vi "Node_ID_AlarmErrors.vi"(11 "error in":errorcluster) -> (4 "transposed array":string[][](array[string]), 6 "Node ID":string[](array[string]), 10 "Name":string[](array[string]), 12 "node RU":T1[](array[typedef]), 13 "node RU 2":T1[](array[typedef]), 14 "node RU 3":string[](array[string]), 15 "error out":errorcluster)   [LabVIEW 2019]
uses:
  <vilib>/OPCUA/controls/NodeId.ctl
panel:
  out "output array":T1[](array[typedef])
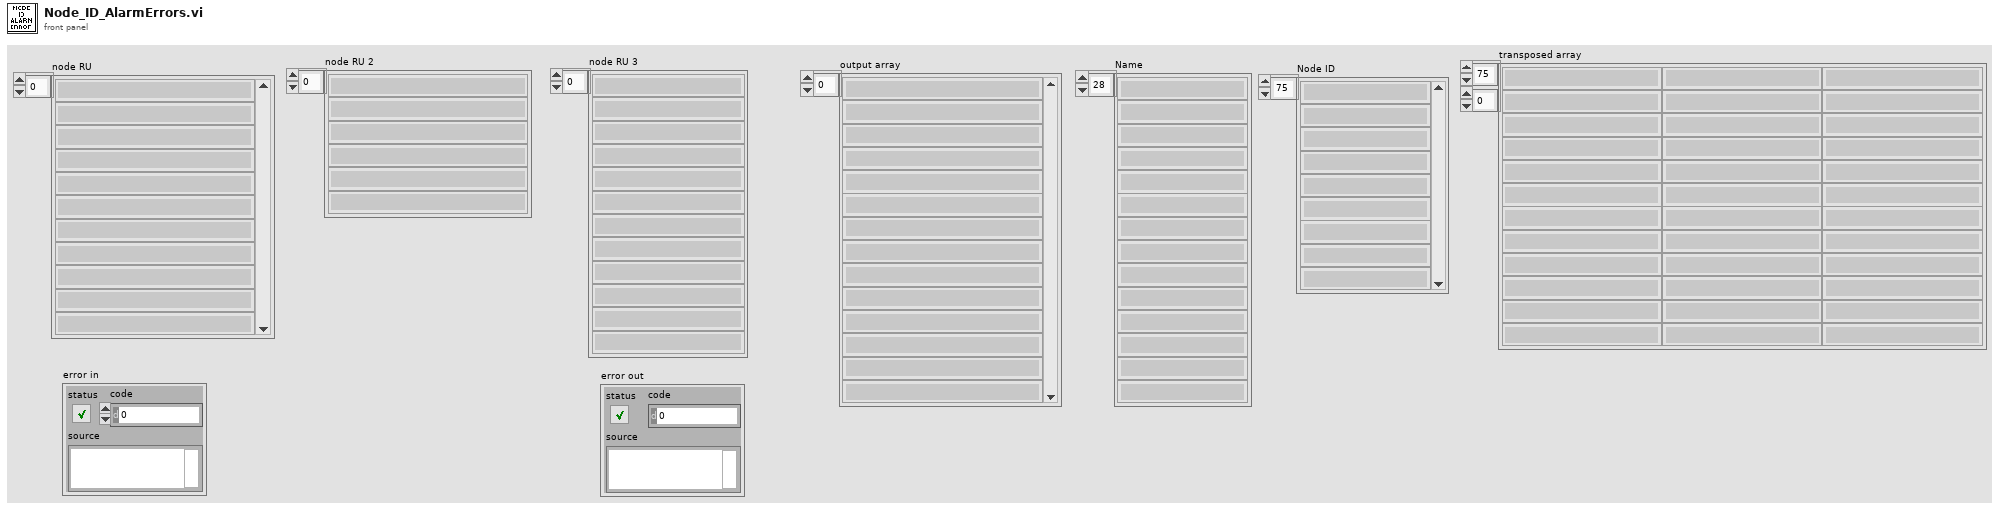
[diagram p1: front panel]
types:
  T1 = typedef "NodeId.ctl" = string
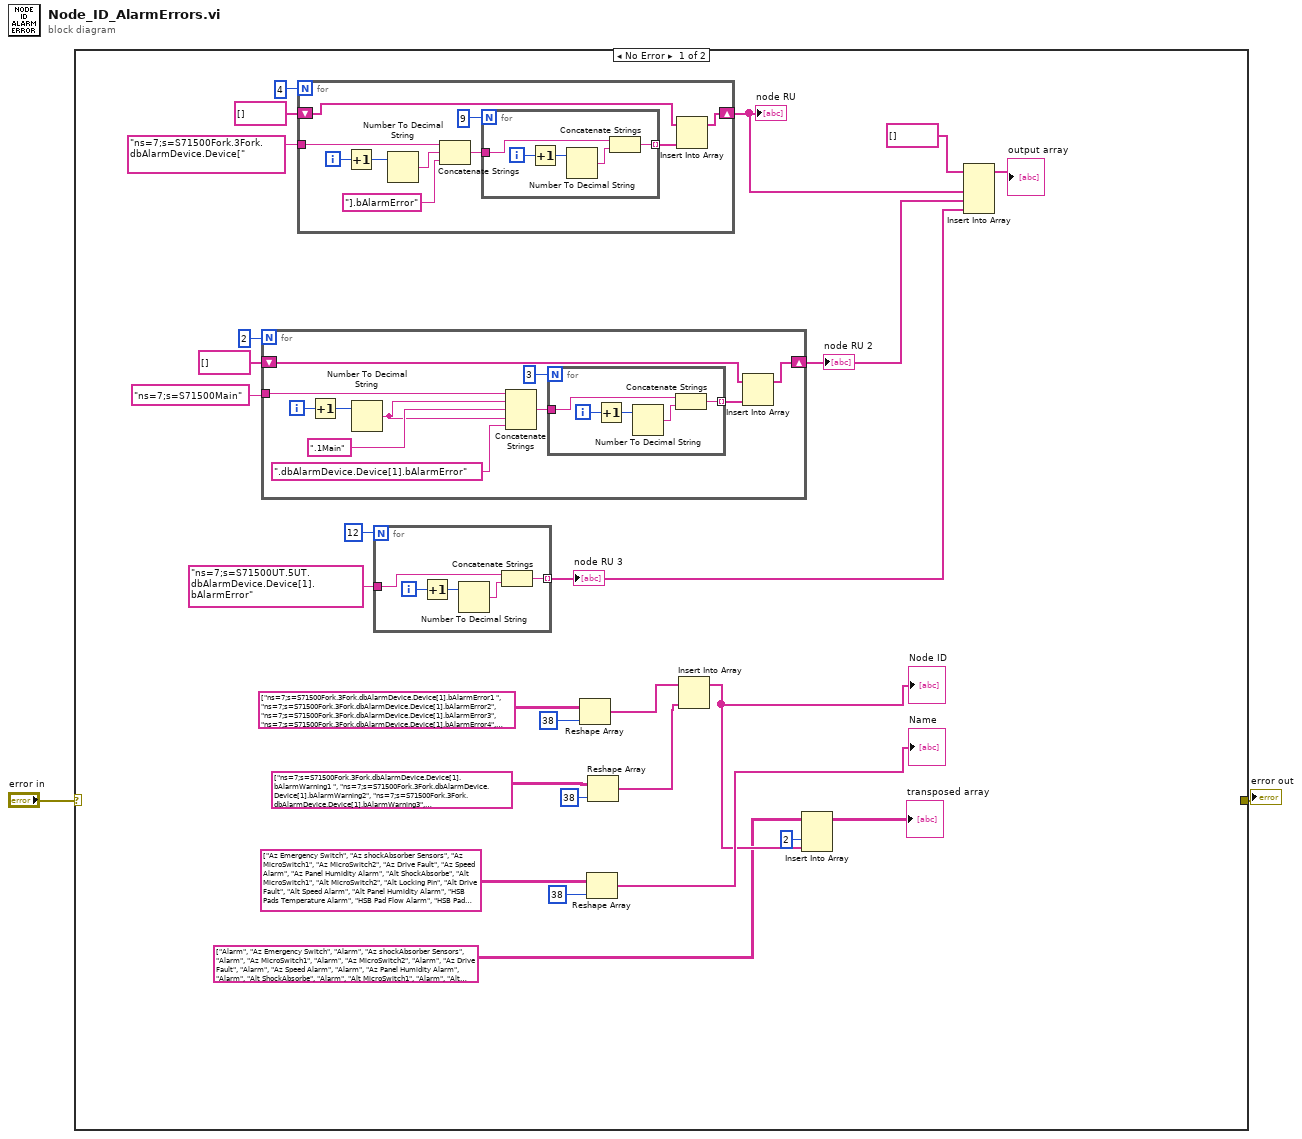
[diagram p0: block diagram]
diagram:
  n1 = case shown="No Error" "error in" {
    selector: "error in" -> [_ w65]
    tunnel: [_ w65] -> w1
    frame No Error {
      n2 = for {
        N: 2 -> [_]
        tunnel: T1 "ns=7;s=S71500Main" ("node RU") -> [w43]
        shift-right: [w40] -> w18
        shift-left: T1[] [] ("node RU") -> [w38]
        i -> [w42]
        n3 = Increment(x=w42) -> (x+1=w44:i32)
        n4 = Number To Decimal String(number=w44) -> (decimal integer string=w36:string)  [unwired: 1 in]
        n5 = Concatenate Strings(w43, w36, ".1Main" ("string"), w36, ".dbAlarmDevice.Device[1].bAlarmError" ("string")) -> (w41:string)
        n6 = for {
          N: 3 -> [_]
          tunnel: w41 -> [w49]
          tunnel: [w45] -> w39 mode=indexing
          i -> [w48]
          n7 = Increment(x=w48) -> (x+1=w47:i32)
          n8 = Number To Decimal String(number=w47) -> (decimal integer string=w46:string)  [unwired: 1 in]
          n9 = Concatenate Strings(w49, w46) -> (w45:string)
        }
        n10 = Insert Into Array(array=w38, new element=w39) -> (w40:T1[])  [unwired: 1 in]
      }
      "node RU 2" <- w18
      n11 = for {
        N: 4 -> [_]
        tunnel: T1 "ns=7;s=S71500Fork.3Fork.dbAlarmDevice.Device[" ("node RU") -> [w57]
        shift-right: [w52] -> w19
        shift-left: T1[] [] ("node RU") -> [w50]
        i -> [w56]
        n12 = Increment(x=w56) -> (x+1=w59:i32)
        n13 = Number To Decimal String(number=w59) -> (decimal integer string=w58:string)  [unwired: 1 in]
        n14 = Concatenate Strings(w57, w58, "].bAlarmError" ("string")) -> (w53:string)
        n15 = for {
          N: 9 -> [_]
          tunnel: w53 -> [w64]
          tunnel: [w60] -> w51 mode=indexing
          i -> [w63]
          n16 = Increment(x=w63) -> (x+1=w62:i32)
          n17 = Number To Decimal String(number=w62) -> (decimal integer string=w61:string)  [unwired: 1 in]
          n18 = Concatenate Strings(w64, w61) -> (w60:string)
        }
        n19 = Insert Into Array(array=w50, new element=w51) -> (w52:T1[])  [unwired: 1 in]
      }
      "node RU" <- w19
      n20 = for {
        N: 12 -> [_]
        tunnel: T1 "ns=7;s=S71500UT.5UT.dbAlarmDevice.Device[1].bAlarmError" ("node RU") -> [w33]
        tunnel: [w29] -> w17 mode=indexing
        i -> [w32]
        n21 = Increment(x=w32) -> (x+1=w31:i32)
        n22 = Number To Decimal String(number=w31) -> (decimal integer string=w30:string)  [unwired: 1 in]
        n23 = Concatenate Strings(w33, w30) -> (w29:string)
      }
      "node RU 3" <- w17
      n24 = Reshape Array(string[][] [["ns=7;s=S71500Fork.3Fork.dbAlarmDevice.Device[1].bAlarmError1 "], ["ns=7;s=S71500Fork.3Fork.dbAlarmDevice.Device[1].bAlarmError2"], ["ns=7;s=S71500Fork.3Fork.dbAlarmDevice.Device[1].bAlarmError3"], ["ns=7;s=S71500Fork.3Fork.dbAlarmDevice.Device[1].bAlarmError4"], ["ns=7;s=S71500Fork.3Fork.dbAlarmDevice.Device[1].bAlarmError6"], ["ns=7;s=S71500Fork.3Fork.dbAlarmDevice.Device[1].bAlarmError7"], ["ns=7;s=S71500Fork.3Fork.dbAlarmDevice.Device[1].bAlarmError8"], ["ns=7;s=S71500Fork.3Fork.dbAlarmDevice.Device[2].bAlarmError2"], ["ns=7;s=S71500Fork.3Fork.dbAlarmDevice.Device[2].bAlarmError3"], ["ns=7;s=S71500Fork.3Fork.dbAlarmDevice.Device[2].bAlarmError4"], ["ns=7;s=S71500Fork.3Fork.dbAlarmDevice.Device[2].bAlarmError5"], ["ns=7;s=S71500Fork.3Fork.dbAlarmDevice.Device[2].bAlarmError6"], ["ns=7;s=S71500Fork.3Fork.dbAlarmDevice.Device[2].bAlarmError7"], ["ns=7;s=S71500Fork.3Fork.dbAlarmDevice.Device[2].bAlarmError8"], ["ns=7;s=S71500Fork.3Fork.dbAlarmDevice.Device[3].bAlarmError2"], ["ns=7;s=S71500Fork.3Fork.dbAlarmDevice.Device[3].bAlarmError3"], ["ns=7;s=S71500Fork.3Fork.dbAlarmDevice.Device[3].bAlarmError4"], ["ns=7;s=S71500Fork.3Fork.dbAlarmDevice.Device[3].bAlarmError5"], ["ns=7;s=S71500Fork.3Fork.dbAlarmDevice.Device[4].bAlarmError8"], ["ns=7;s=S71500Fork.3Fork.dbAlarmDevice.Device[4].bAlarmError9"], ["ns=7;s=S71500Main1.1Main1.dbAlarmDevice.Device[1].bAlarmError1 "], ["ns=7;s=S71500Main1.1Main1.dbAlarmDevice.Device[1].bAlarmError2"], ["ns=7;s=S71500Main1.1Main1.dbAlarmDevice.Device[1].bAlarmError3"], ["ns=7;s=S71500Main2.1Main2.dbAlarmDevice.Device[1].bAlarmError1 "], ["ns=7;s=S71500Main2.1Main2.dbAlarmDevice.Device[1].bAlarmError2"], ["ns=7;s=S71500Main2.1Main2.dbAlarmDevice.Device[1].bAlarmError3"], ["ns=7;s=S71500UT.5UT.dbAlarmDevice.Device[1].bAlarmError1"], ["ns=7;s=S71500UT.5UT.dbAlarmDevice.Device[1].bAlarmError2"], ["ns=7;s=S71500UT.5UT.dbAlarmDevice.Device[1].bAlarmError3"], ["ns=7;s=S71500UT.5UT.dbAlarmDevice.Device[1].bAlarmError4"], ["ns=7;s=S71500UT.5UT.dbAlarmDevice.Device[1].bAlarmError5"], ["ns=7;s=S71500UT.5UT.dbAlarmDevice.Device[1].bAlarmError6"], ["ns=7;s=S71500UT.5UT.dbAlarmDevice.Device[1].bAlarmError7"], ["ns=7;s=S71500UT.5UT.dbAlarmDevice.Device[1].bAlarmError8"], ["ns=7;s=S71500UT.5UT.dbAlarmDevice.Device[1].bAlarmError9"], ["ns=7;s=S71500UT.5UT.dbAlarmDevice.Device[1].bAlarmError10"], ["ns=7;s=S71500UT.5UT.dbAlarmDevice.Device[1].bAlarmError11"], ["ns=7;s=S71500UT.5UT.dbAlarmDevice.Device[1].bAlarmError12"]] ("data"), 38 ("dimension size")) -> (w6:string[])
      n25 = Reshape Array(string[][] [["Az Emergency Switch"], ["Az shockAbsorber Sensors"], ["Az MicroSwitch1"], ["Az MicroSwitch2"], ["Az Drive Fault"], ["Az Speed Alarm"], ["Az Panel Humidity Alarm"], ["Alt ShockAbsorbe"], ["Alt MicroSwitch1"], ["Alt MicroSwitch2"], ["Alt Locking Pin"], ["Alt Drive Fault"], ["Alt Speed Alarm"], ["Alt Panel Humidity Alarm"], ["HSB Pads Temperature Alarm"], ["HSB Pad Flow Alarm"], ["HSB Pad Pressure Alarm"], ["HSB Pads Filters Alarm"], ["Fork Panel Humidity Alarm"], ["Fork Panel Temperator Alarm"], ["Main Emergency Microswitch"], ["UPS Input Alarm"], ["UPS Output Alarm"], ["Main Emergency Microswitch"], ["UPS Input Alarm"], ["UPS Output Alarm"], ["HSB Emergency Alarm"], ["Feed Over Pressure Alarm"], ["Accumulator Pressure Alarm"], ["Main And Reserve Pressure Alarm"], ["HSB Pad Inside Pressure Alarm"], ["HSB Filter Alarm"], ["Oil Level Alarm"], ["Pressure Switch Alarm"], ["Feeds Alarm"], ["UT Panel Humidity Alarm"], ["UT Panel Temperator Alarm"], ["Feed Under Pressure Alarm"]] ("data"), 38 ("dimension size")) -> (→"Name":string[])
      n26 = Reshape Array(string[][] [["ns=7;s=S71500Fork.3Fork.dbAlarmDevice.Device[1].bAlarmWarning1 "], ["ns=7;s=S71500Fork.3Fork.dbAlarmDevice.Device[1].bAlarmWarning2"], ["ns=7;s=S71500Fork.3Fork.dbAlarmDevice.Device[1].bAlarmWarning3"], ["ns=7;s=S71500Fork.3Fork.dbAlarmDevice.Device[1].bAlarmWarning4"], ["ns=7;s=S71500Fork.3Fork.dbAlarmDevice.Device[1].bAlarmWarning6"], ["ns=7;s=S71500Fork.3Fork.dbAlarmDevice.Device[1].bAlarmWarning7"], ["ns=7;s=S71500Fork.3Fork.dbAlarmDevice.Device[1].bAlarmWarning8"], ["ns=7;s=S71500Fork.3Fork.dbAlarmDevice.Device[2].bAlarmWarning2"], ["ns=7;s=S71500Fork.3Fork.dbAlarmDevice.Device[2].bAlarmWarning3"], ["ns=7;s=S71500Fork.3Fork.dbAlarmDevice.Device[2].bAlarmWarning4"], ["ns=7;s=S71500Fork.3Fork.dbAlarmDevice.Device[2].bAlarmWarning5"], ["ns=7;s=S71500Fork.3Fork.dbAlarmDevice.Device[2].bAlarmWarning6"], ["ns=7;s=S71500Fork.3Fork.dbAlarmDevice.Device[2].bAlarmWarning7"], ["ns=7;s=S71500Fork.3Fork.dbAlarmDevice.Device[2].bAlarmWarning8"], ["ns=7;s=S71500Fork.3Fork.dbAlarmDevice.Device[3].bAlarmWarning2"], ["ns=7;s=S71500Fork.3Fork.dbAlarmDevice.Device[3].bAlarmWarning3"], ["ns=7;s=S71500Fork.3Fork.dbAlarmDevice.Device[3].bAlarmWarning4"], ["ns=7;s=S71500Fork.3Fork.dbAlarmDevice.Device[3].bAlarmWarning5"], ["ns=7;s=S71500Fork.3Fork.dbAlarmDevice.Device[4].bAlarmWarning8"], ["ns=7;s=S71500Fork.3Fork.dbAlarmDevice.Device[4].bAlarmWarning9"], ["ns=7;s=S71500Main1.1Main1.dbAlarmDevice.Device[1].bAlarmWarning1 "], ["ns=7;s=S71500Main1.1Main1.dbAlarmDevice.Device[1].bAlarmWarning2"], ["ns=7;s=S71500Main1.1Main1.dbAlarmDevice.Device[1].bAlarmWarning3"], ["ns=7;s=S71500Main2.1Main2.dbAlarmDevice.Device[1].bAlarmWarning1 "], ["ns=7;s=S71500Main2.1Main2.dbAlarmDevice.Device[1].bAlarmWarning2"], ["ns=7;s=S71500Main2.1Main2.dbAlarmDevice.Device[1].bAlarmWarning3"], ["ns=7;s=S71500UT.5UT.dbAlarmDevice.Device[1].bAlarmWarning1"], ["ns=7;s=S71500UT.5UT.dbAlarmDevice.Device[1].bAlarmWarning2"], ["ns=7;s=S71500UT.5UT.dbAlarmDevice.Device[1].bAlarmWarning3"], ["ns=7;s=S71500UT.5UT.dbAlarmDevice.Device[1].bAlarmWarning4"], ["ns=7;s=S71500UT.5UT.dbAlarmDevice.Device[1].bAlarmWarning5"], ["ns=7;s=S71500UT.5UT.dbAlarmDevice.Device[1].bAlarmWarning6"], ["ns=7;s=S71500UT.5UT.dbAlarmDevice.Device[1].bAlarmWarning7"], ["ns=7;s=S71500UT.5UT.dbAlarmDevice.Device[1].bAlarmWarning8"], ["ns=7;s=S71500UT.5UT.dbAlarmDevice.Device[1].bAlarmWarning9"], ["ns=7;s=S71500UT.5UT.dbAlarmDevice.Device[1].bAlarmWarning10"], ["ns=7;s=S71500UT.5UT.dbAlarmDevice.Device[1].bAlarmWarning11"], ["ns=7;s=S71500UT.5UT.dbAlarmDevice.Device[1].bAlarmWarning12"]] ("data"), 38 ("dimension size")) -> (w5:string[])
      n27 = Insert Into Array(array=w6, new element=w5) -> (w4:string[])  [unwired: 1 in]
      "Node ID" <- w4
      n28 = Insert Into Array(array=string[][] [["Alarm", "Az Emergency Switch"], ["Alarm", "Az shockAbsorber Sensors"], ["Alarm", "Az MicroSwitch1"], ["Alarm", "Az MicroSwitch2"], ["Alarm", "Az Drive Fault"], ["Alarm", "Az Speed Alarm"], ["Alarm", "Az Panel Humidity Alarm"], ["Alarm", "Alt ShockAbsorbe"], ["Alarm", "Alt MicroSwitch1"], ["Alarm", "Alt MicroSwitch2"], ["Alarm", "Alt Locking Pin"], ["Alarm", "Alt Drive Fault"], ["Alarm", "Alt Speed Alarm"], ["Alarm", "Alt Panel Humidity Alarm"], ["Alarm", "HSB Pads Temperature Alarm"], ["Alarm", "HSB Pad Flow Alarm"], ["Alarm", "HSB Pad Pressure Alarm"], ["Alarm", "HSB Pads Filters Alarm"], ["Alarm", "Fork Panel Humidity Alarm"], ["Alarm", "Fork Panel Temperator Alarm"], ["Alarm", "Main Emergency Microswitch"], ["Alarm", "UPS Input Alarm"], ["Alarm", "UPS Output Alarm"], ["Alarm", "Main Emergency Microswitch"], ["Alarm", "UPS Input Alarm"], ["Alarm", "UPS Output Alarm"], ["Alarm", "HSB Emergency Alarm"], ["Alarm", "Feed Over Pressure Alarm"], ["Alarm", "Accumulator Pressure Alarm"], ["Alarm", "Main And Reserve Pressure Alarm"], ["Alarm", "HSB Pad Inside Pressure Alarm"], ["Alarm", "HSB Filter Alarm"], ["Alarm", "Oil Level Alarm"], ["Alarm", "Pressure Switch Alarm"], ["Alarm", "Feeds Alarm"], ["Alarm", "UT Panel Humidity Alarm"], ["Alarm", "UT Panel Temperator Alarm"], ["Alarm", "Feed Under Pressure Alarm"], ["Warning", "Az Emergency Switch"], ["Warning", "Az shockAbsorber Sensors"], ["Warning", "Az MicroSwitch1"], ["Warning", "Az MicroSwitch2"], ["Warning", "Az Drive Fault"], ["Warning", "Az Speed Alarm"], ["Warning", "Az Panel Humidity Alarm"], ["Warning", "Alt ShockAbsorbe"], ["Warning", "Alt MicroSwitch1"], ["Warning", "Alt MicroSwitch2"], ["Warning", "Alt Locking Pin"], ["Warning", "Alt Drive Fault"], ["Warning", "Alt Speed Alarm"], ["Warning", "Alt Panel Humidity Alarm"], ["Warning", "HSB Pads Temperature Alarm"], ["Warning", "HSB Pad Flow Alarm"], ["Warning", "HSB Pad Pressure Alarm"], ["Warning", "HSB Pads Filters Alarm"], ["Warning", "Fork Panel Humidity Alarm"], ["Warning", "Fork Panel Temperator Alarm"], ["Warning", "Main Emergency Microswitch"], ["Warning", "UPS Input Alarm"], ["Warning", "UPS Output Alarm"], ["Warning", "Main Emergency Microswitch"], ["Warning", "UPS Input Alarm"], ["Warning", "UPS Output Alarm"], ["Warning", "HSB Emergency Alarm"], ["Warning", "Feed Over Pressure Alarm"], ["Warning", "Accumulator Pressure Alarm"], ["Warning", "Main And Reserve Pressure Alarm"], ["Warning", "HSB Pad Inside Pressure Alarm"], ["Warning", "HSB Filter Alarm"], ["Warning", "Oil Level Alarm"], ["Warning", "Pressure Switch Alarm"], ["Warning", "Feeds Alarm"], ["Warning", "UT Panel Humidity Alarm"], ["Warning", "UT Panel Temperator Alarm"], ["Warning", "Feed Under Pressure Alarm"]] ("data"), index (col)=2 ("disabled index (col)"), new element=w4) -> (→"transposed array":string[][])  [unwired: 1 in]
      n29 = Insert Into Array(array=T1[] [] ("node RU"), new element #1=w19, new element #2=w18, new element #3=w17) -> (→"output array":T1[])  [unwired: 1 in]
    }
    frame Error {
    }
  }
  "error out" <- w1
